vi "Page.Set.vi"(8 "error in (no error)":errorcluster, 10 "message value":string, 11 "State Variables":T1) -> (0 "error out":errorcluster, 3 "State Variables":T1)   [LabVIEW 2015, in "Station.Execution.lvlib"]
uses:
  Station.Execution.lvlib
  Types/Main.StateVariables.ctl
  <vilib>/Utility/miscctls.llb/LVPositionTypeDef.ctl
  Types/Execute.UserEventRefs.ctl
  <vilib>/NI Veristand/Execution/Workspace/SystemStateRegEventRef.ctl
  <vilib>/NI Veristand/Execution/Workspace/Target State Info.ctl
  <vilib>/NI Veristand/Execution/Workspace/Target State.ctl
  <vilib>/NI Veristand/Execution/WaveformStreaming/Waveform Data Watcher Event Data (DBL).ctl
  <vilib>/NI Veristand/Execution/WaveformStreaming/WaveformStreamSpecification.ctl
  NationalInstruments.VeriStand.ClientAPI
  <vilib>/NI Veristand/Execution/Workspace/SystemStateEventRef.ctl
  <vilib>/NI Veristand/Execution/Workspace/WorkspaceAPI.ctl
  Types/UI.Object.ctl
  Types/Waveforms.Info.ctl
  <vilib>/NI Veristand/Execution/WaveformStreaming/Registered Waveform Streams Data Event Refnum (DBL).ctl
  <vilib>/NI Veristand/Execution/WaveformStreaming/WaveformDataWatcherDBL.ctl
  <vilib>/NI Veristand/Execution/WaveformStreaming/WaveformStreamingAPI.ctl
  <vilib>/NI Veristand/Execution/Workspace/NI_VS Workspace ExecutionAPI.lvlib
  <vilib>/NI Veristand/Execution/WaveformStreaming/NI_VS Waveform Streaming Interface.lvlib
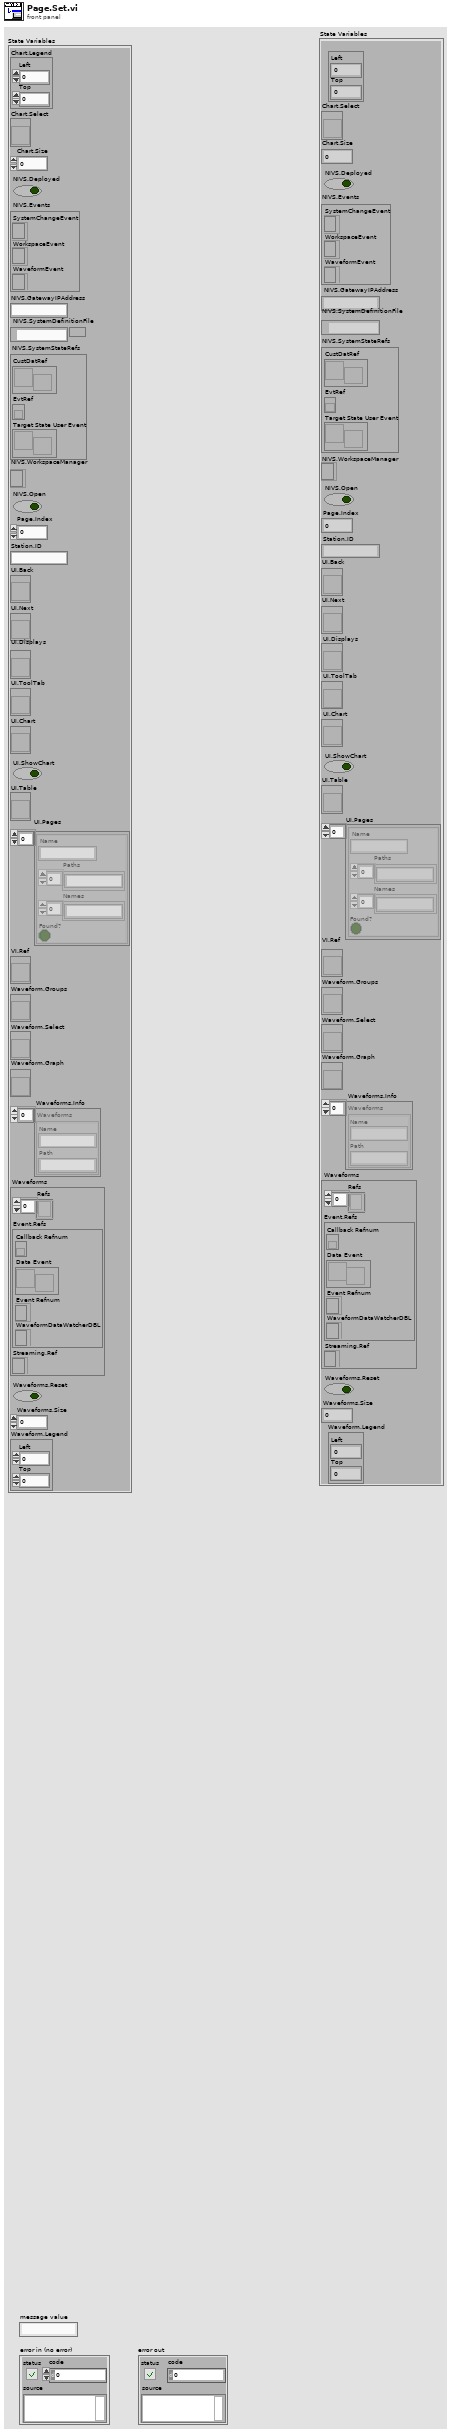
[diagram p1: front panel]
types:
  T1 = typedef "Station.Execution.lvlib/Main.StateVariables.ctl" = cluster{"Chart.Legend":T2, "Chart.Select":refnum<vi>, "Chart.Size":i32, "NIVS.Deployed":bool, "NIVS.Events":T3, "NIVS.GatewayIPAddress":string, "NIVS.SystemDefinitionFile":path, "NIVS.SystemStateRefs":T5, "NIVS.WorkspaceManager":T6, "NIVS.Open":bool, "Page.Index":u32, "Station.ID":string, "UI.Back":refnum<vi>, "UI.Next":refnum<vi>, "UI.Displays":refnum<vi>, "UI.ToolTab":refnum<vi>, "UI.Chart":refnum<vi>, "UI.ShowChart":bool, "UI.Table":refnum<vi>, "UI.Pages":T7[], "VI.Ref":refnum<vi>, "Waveform.Groups":refnum<vi>, "Waveform.Select":refnum<vi>, "Waveform.Graph":refnum<vi>, "Waveforms.Info":T8[], "Waveforms":cluster{"Refs":T9[], "Event.Refs":T10, "Streaming.Ref":T12}, "Waveforms.Reset":bool, "Waveforms.Size":i32, "Waveform.Legend":T2}
  T2 = typedef "LVPositionTypeDef.ctl" = cluster{"Left":i32, "Top":i32}
  T3 = typedef "Station.Execution.lvlib/Execute.UserEventRefs.ctl" = cluster{"SystemChangeEvent":T4, "WorkspaceEvent":refnum<event-registration>, "WaveformEvent":refnum<event-registration>}
  T4 = typedef "NI_VS Workspace ExecutionAPI.lvlib/SystemStateRegEventRef.ctl" = refnum<event-registration>
  T5 = typedef "NI_VS Workspace ExecutionAPI.lvlib/SystemStateEventRef.ctl" = cluster{"CustDatRef":refnum<user-event>, "EvtRef":refnum<k27>, "Target State User Event":refnum<user-event>}
  T6 = typedef "NI_VS Workspace ExecutionAPI.lvlib/WorkspaceAPI.ctl" = refnum<k24>
  T7 = typedef "Station.Execution.lvlib/UI.Object.ctl" = cluster{"Name":string, "Paths":string[], "Names":string[], "Found?":bool}
  T8 = typedef "Station.Execution.lvlib/Waveforms.Info.ctl" = cluster{"Name":string, "Path":string}
  T9 = typedef "NI_VS Waveform Streaming Interface.lvlib/WaveformStreamSpecification.ctl" = refnum<k24>
  T10 = typedef "NI_VS Waveform Streaming Interface.lvlib/Registered Waveform Streams Data Event Refnum (DBL).ctl" = cluster{"Callback Refnum":refnum<k27>, "Data Event":refnum<user-event>, "Event Refnum":refnum<event-registration>, "WaveformDataWatcherDBL":T11}
  T11 = typedef "NI_VS Waveform Streaming Interface.lvlib/WaveformDataWatcherDBL.ctl" = refnum<k24>
  T12 = typedef "NI_VS Waveform Streaming Interface.lvlib/WaveformStreamingAPI.ctl" = refnum<k24>
  T13 = enum8{"Enabled", "Disabled", "Disabled and Grayed Out"}
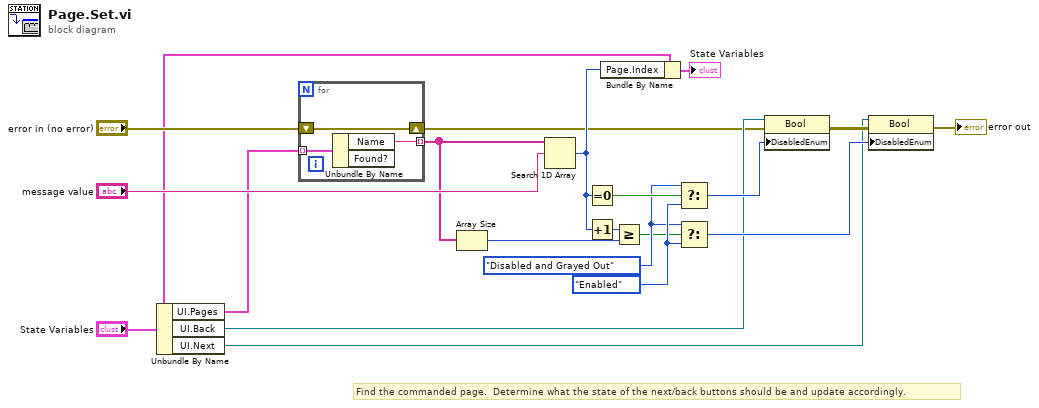
[diagram p0: block diagram]
diagram:
  w16 = T13."Enabled" ("f")
  w15 = T13."Disabled and Grayed Out" ("Disabled")
  # "Find the commanded page.  Determine what the state of the next/back buttons should be and update accordingly."
  n1 = Unbundle By Name("State Variables") -> ("UI.Pages"=w7:T7[], "UI.Back"=w8:refnum<vi>, "UI.Next"=w9:refnum<vi>)
  n2 = for {
    tunnel: w7 -> [w23] mode=indexing
    tunnel: [w22] -> w1 mode=indexing
    shift-right: [w21] -> w3
    shift-left: "error in (no error)" -> [w21]
    n3 = Unbundle By Name(w23) -> ("Name"=w22:string)  [unwired: 1 out]
  }
  n4 = Array Size(array=w1) -> (size(s)=w13:i32)
  n5 = Search 1D Array(1D array=w1, element="message value") -> (index of element=w4:i32)  [unwired: 1 in]
  n6 = Equal To 0?(x=w4) -> (x = 0?=w18:bool)
  n7 = Increment(x=w4) -> (x+1=w12:i32)
  n8 = Bundle By Name(cluster="State Variables", "Page.Index"=w4) -> (→"State Variables":T1)
  n9 = Greater Or Equal?(x=w12, y=w13) -> (x >= y?=w11:bool)
  n10 = Select(t=w15, s=w18, f=w16) -> (s? t:f=w17:T13)
  n11 = Select(t=w15, s=w11, f=w16) -> (s? t:f=w14:T13)
  n12 = property class="Bool"(reference=w8, error in=w3, "DisabledEnum"=w17) -> (error out=w19:errorcluster)  [unwired: 1 out]
  n13 = property class="Bool"(reference=w9, error in=w19, "DisabledEnum"=w14) -> (error out=→"error out":errorcluster)  [unwired: 1 out]
